vi "Read Selection Colors.vi"(8 "error in (no error)":errorcluster, 11 "Panel Object in":refnum<class "Panel Object.lvclass">) -> (0 "error out":errorcluster, 2 "Selection Colors":T1={"Normal"=13816530, "Mouse-over"=0, "Selected"=9868950, "Selected Mouse-over"=9868950}, 3 "Panel Object out":refnum<class "Panel Object.lvclass">)   [LabVIEW 2017, in "Panel Object.lvclass"]
uses:
  Panel Object.lvclass
  Typedefs/Selection Colors--Cluster.ctl
  Panel Object.lvclass/Panel Object.ctl
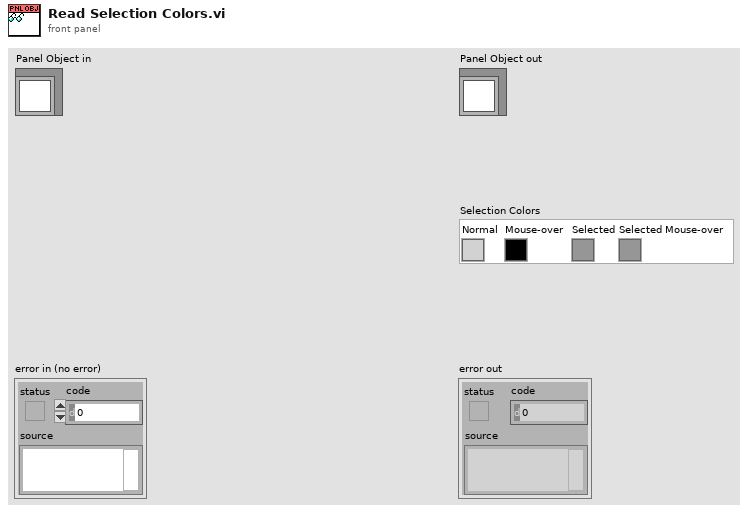
[diagram p1: front panel]
types:
  T1 = typedef "Selection Colors--Cluster.ctl" = cluster{"Normal":u32, "Mouse-over":u32, "Selected":u32, "Selected Mouse-over":u32}
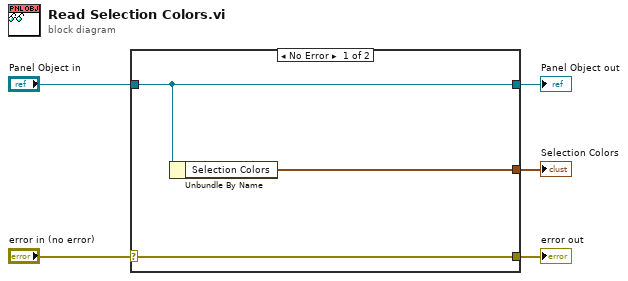
[diagram p0: block diagram]
diagram:
  n1 = case shown="No Error" "error in (no error)" {
    selector: "error in (no error)" -> [w8 w9]
    tunnel: [w8 w9] -> w4
    tunnel: [w7 w10] -> w2
    tunnel: "Panel Object in" -> [w7 w10]
    tunnel: [w6 _] -> w1
    frame No Error {
      n2 = Unbundle By Name(w7) -> ("Selection Colors"=w6:T1)
    }
    frame Error {
    }
  }
  "error out" <- w4
  "Panel Object out" <- w2
  "Selection Colors" <- w1
